vi "Ctor.vi"(8 "error in (no error)":errorcluster, 10 "SQLite":refnum<class "SQLite.lvclass">) -> (0 "error out":errorcluster, 3 "Submission DB out":refnum<class "Submission DB.lvclass">)   [LabVIEW 2020, in "Summer of LabVIEW.lvlib" / "Submission DB.lvclass"]
uses:
  Submission DB.lvclass
  SQLite/SQLite.lvclass
  Submission DB.lvclass/Submission DB.ctl
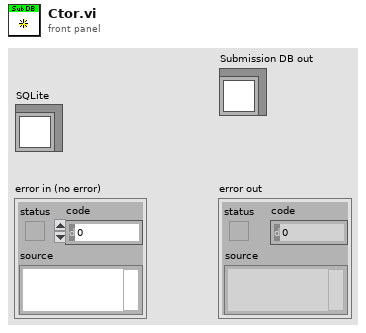
[diagram p1: front panel]
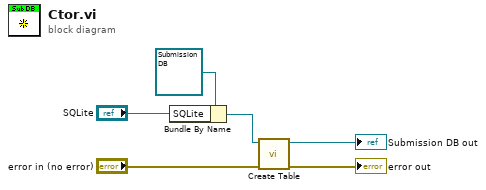
[diagram p0: block diagram]
diagram:
  n1 = Bundle By Name(cluster=refnum<class "Submission DB.lvclass"> refnum ("Submission DB in"), "SQLite"="SQLite") -> (w1:refnum<class "Submission DB.lvclass">)
  n2 = call "Create Table.vi"("error in (no error)"="error in (no error)", "Submission DB in"=w1) -> ("error out"=→"error out":errorcluster, "Submission DB out"=→"Submission DB out":refnum<class "Submission DB.lvclass">)  [unwired: 8 in]
